vi "Ignore 1073676294 Error.vi"(8 "error in (no error)":errorcluster) -> (0 "error out":errorcluster)   [LabVIEW 2020]
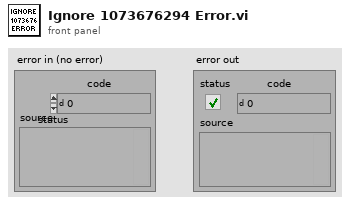
[diagram p1: front panel]
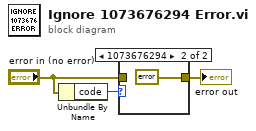
[diagram p0: block diagram]
diagram:
  n1 = Unbundle By Name("error in (no error)") -> ("code"=w3:i32)
  n2 = case shown="1073676294" w3 {
    tunnel: [w4 errorcluster {"status"=FALSE, "code"=0, "source"=""} ("error constant")] -> w2
    tunnel: "error in (no error)" -> [w4 _]
    frame 0, Default {
    }
    frame 1073676294 {
    }
  }
  "error out" <- w2
